vi "Degrees to Radians (Scalar DBL).vi"(3 "angle (deg)":dbl caption="角（角度）") -> (1 "angle (rad)":dbl caption="角（弧度）")   [LabVIEW 2011, in "NI_AngleManipulation.lvlib"]
doc: "Converts an angle from degrees to radians."
uses:
  <vilib>/Utility/AngleManip/NI_AngleManipulation.lvlib
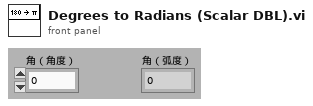
[diagram p1: front panel]
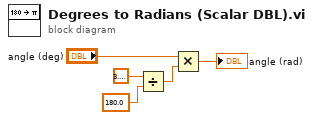
[diagram p0: block diagram]
diagram:
  n1 = Divide(x=3.141592653589793, y=180.0) -> (x/y=w2:dbl)
  n2 = Multiply(x="angle (deg)", y=w2) -> (x*y=→"angle (rad)":dbl)
